vi "Load Wave File Data.vi"(10 "prompt":string="Open Tachometer Wav File", 11 "start path":path) -> (0 "cancelled":bool, 1 "sound format":T1, 2 "data":i16[](array[numeric]), 3 "wave file path out":path)   [LabVIEW 2017]
uses:
  <vilib>/addons/Sound and Vibration/Order Analysis/Example Support/Demo VI/Start-Up Kit/File Access/Sound Format+.ctl
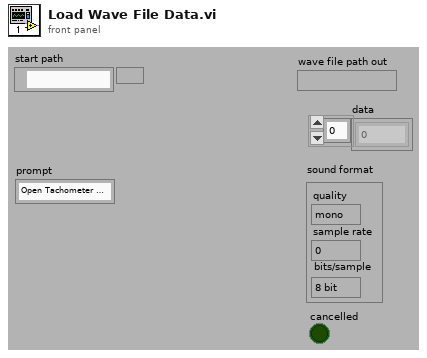
[diagram p1: front panel]
types:
  T1 = typedef "Sound Format+.ctl" = cluster{"quality":enum16{"mono", "stereo"}, "sample rate":u32, "bits/sample":enum16{"8 bit", "16 bit"}}
  T2 = enum32{"existing file", "new file", "new or existing file", "existing dir", "new dir", "new or existing dir", "existing file (use LLBs)", "new file (use LLBs)", "new or existing file (use LLBs)", "new or existing file or directory (use LLBs)"}
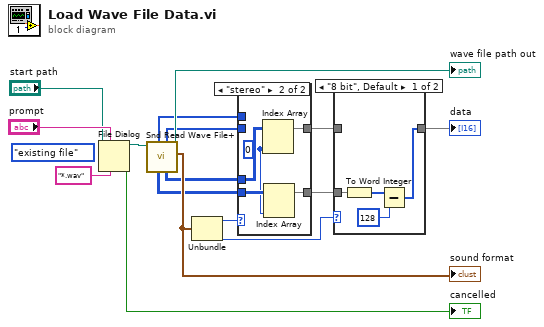
[diagram p0: block diagram]
diagram:
  (unwired) T2."existing file" ("select mode (2)")
  n1 = File Dialog(6:"*.wav" ("pattern"), 7:"prompt", 11:"start path") -> (1:→"cancelled":bool, 3:w12:path)  [unwired: 4 in, 2 out]
  n2 = call <vilib>:"Snd Read Wave File+.vi"("wave file path"=w12) -> ("sound format"=w10:T1, "wave file path out"=→"wave file path out":path, "stereo 16-bit"=w6:i16[][], "mono 16-bit"=w7:i16[], "stereo 8-bit"=w5:u8[][], "mono 8-bit"=w8:u8[])  [unwired: 4 in, 1 out]
  "sound format" <- w10
  n3 = Unbundle(w10) -> ("quality"=w9:enum16{"mono", "stereo"}, "bits/sample"=w3:enum16{"8 bit", "16 bit"})  [unwired: 1 out]
  n4 = case shown="\"stereo\"" w9 {
    tunnel: w8 -> [w17 _]
    tunnel: w7 -> [w18 _]
    tunnel: w6 -> [_ w23]
    tunnel: w5 -> [_ w22]
    tunnel: [w18 w21] -> w4
    tunnel: [w17 w20] -> w2
    frame "mono", Default {
    }
    frame "stereo" {
      w19 = 0 ("Disabled Index (col)")
      n5 = Index Array(array=w23, index (col)=w19) -> (element=w21:i16[])  [unwired: 1 in]
      n6 = Index Array(array=w22, index (col)=w19) -> (element=w20:u8[])  [unwired: 1 in]
    }
  }
  n7 = case shown="\"8 bit\", Default" w3 {
    tunnel: w4 -> [_ w28]
    tunnel: [w26 w28] -> w1
    tunnel: w2 -> [w27 _]
    frame "8 bit", Default {
      n8 = To Word Integer(number=w27) -> (16bit integer=w25:i16[])
      n9 = Subtract(x=w25, y=i16 128) -> (x-y=w26:i16[])
    }
    frame "16 bit" {
    }
  }
  "data" <- w1
